vi "ReadMVC.vi"() -> ()   [LabVIEW 2014]
panel:
  in  "stop":bool
  out "Actual Force (White)":dynamicdata(graph) caption="Actual Force (White) and Target (Red)"
  in  "Start of Data Window":dbl(slide) caption="Begin Offset" scale=0.0..1000.0 scale format="%#_2f"
  in  "Length of Data Window":dbl(slide)=20.0 caption="Length" scale=0.0..1000.0
  out "Maximum":dbl
  out "Time of Maximum":dbl format="%#_4g"
  out "Range":dbl format="%#_5g"
  out "Minimum":dbl format="%#_3g"
  out "Time of Minimum":dbl format="%#_4g"
  out "Duration (s)":dbl
  out "Average":dbl
  in  "Measure Now":bool
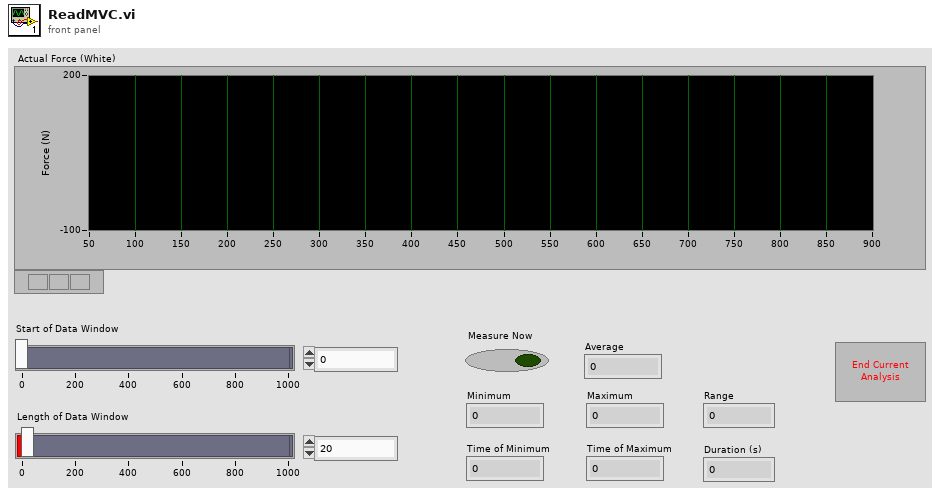
[diagram p1: front panel]
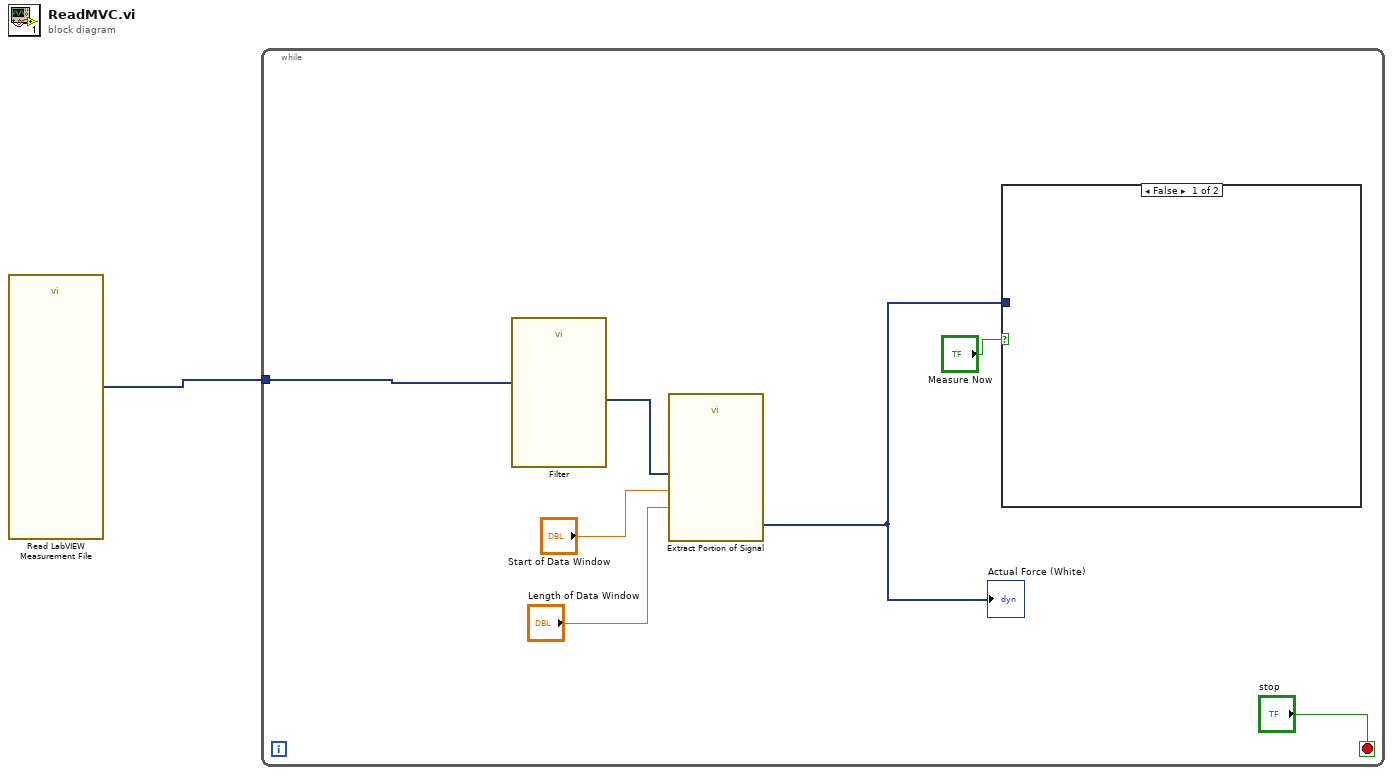
[diagram p0: block diagram]
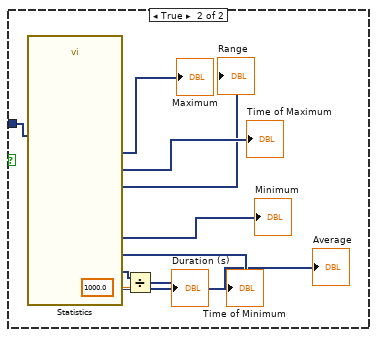
[diagram p2: hidden frame]
diagram:
  n1 = call "Read LabVIEW Measurement File"() -> ("Signals"=w1:dynamicdata)  [unwired: 6 in, 5 out]
  n2 = while {
    tunnel: w1 -> [w2]
    stop <- "stop" stop-if-true
    n3 = call "Filter"("Signal"=w2) -> ("Filtered Signal"=w4:dynamicdata)  [unwired: 9 in, 1 out]
    n4 = call "Extract Portion of Signal"("Length"="Length of Data Window", "Begin Offset"="Start of Data Window", "Signals"=w4) -> ("Section"=w3:dynamicdata)  [unwired: 7 in, 1 out]
    "Actual Force (White)" <- w3
    n5 = case shown="False" "Measure Now" {
      tunnel: w3 -> [_ w13]
      frame False {
      }
      frame True {
        n6 = call "Statistics"("Signals"=w13) -> ("Total Samples"=w10:dynamicdata, "Arithmetic Mean"=→"Average":dynamicdata, "Range"=→"Range":dynamicdata, "Time of Minimum"=→"Time of Minimum":dynamicdata, "Minimum"=→"Minimum":dynamicdata, "Time of Maximum"=→"Time of Maximum":dynamicdata, "Maximum"=→"Maximum":dynamicdata)  [unwired: 19 in, 1 out]
        n7 = Divide(x=w10, y=1000.0) -> (x/y=→"Duration (s)":dynamicdata)
      }
    }
  }
